vi "Timed Message_Stop.vi"(0 "Timed Message In":refnum<class "Timed Message.lvclass">, 11 "error in (no error)":errorcluster) -> (15 "error out":errorcluster)   [LabVIEW 2012, in "Timed Message.lvclass"]
uses:
  Timed Message.lvclass
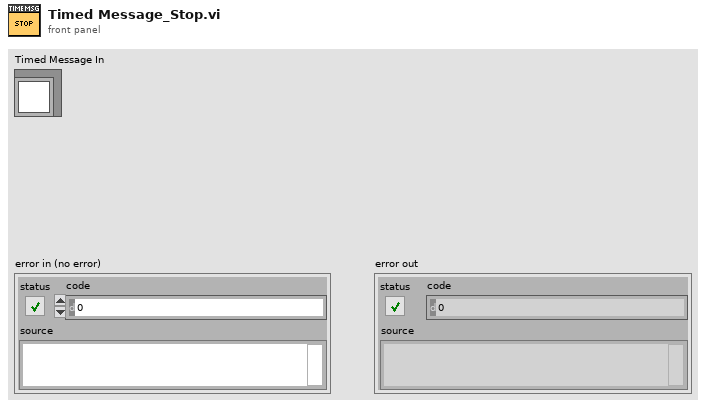
[diagram p1: front panel]
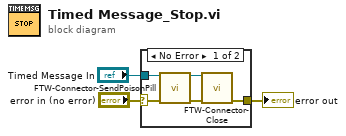
[diagram p0: block diagram]
diagram:
  n1 = case shown="No Error" "error in (no error)" {
    selector: "error in (no error)" -> [w7 w9]
    tunnel: "Timed Message In" -> [w8 _]
    tunnel: [w5 w9] -> w1
    frame No Error {
      n2 = call-dynamic "FTW-Connector-SendPoisonPill.vi"("FTW Actor Connector"=w8, "error in"=w7) -> ("FTW Actor Connector out"=w4:refnum<class "Timed Message.lvclass">, "error out"=w6:errorcluster)  [unwired: 9 in, 3 out]
      n3 = call-dynamic "FTW-Connector-Close.vi"("FTW Actor Connector"=w4, "error in"=w6) -> ("error out"=w5:errorcluster)  [unwired: 13 in]
    }
    frame Error {
    }
  }
  "error out" <- w1
